vi "robot - Tangent Points.vi"(9 "Diameter":dbl, 10 "Rotation":dbl, 11 "Center Point":cluster{"X":dbl, "Y":dbl}) -> (2 "Second Point":cluster{"X":dbl, "Y":dbl}, 3 "First Point":cluster{"X":dbl, "Y":dbl})   [LabVIEW 2016]
doc: "This VI returns the two points at which a diameter perpendicular to the radius at the given angle (in radians) meet the circle defined by center and diameter."
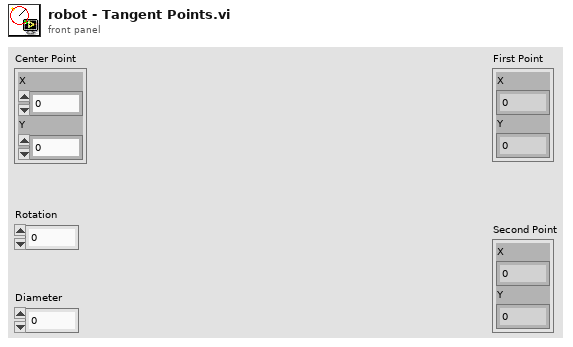
[diagram p1: front panel]
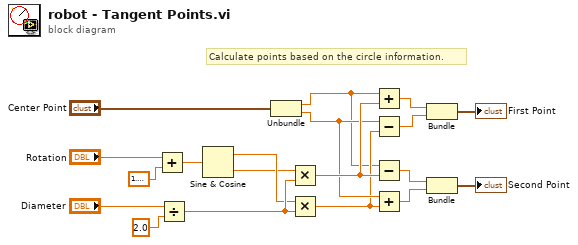
[diagram p0: block diagram]
diagram:
  # "Calculate points based on the circle information."
  n1 = Add(x="Rotation", y=1.5707963267948966) -> (x+y=w16:dbl)
  n2 = Divide(x="Diameter", y=2.0) -> (x/y=w14:dbl)
  n3 = Sine & Cosine(0:w16) -> (1:w13:dbl, 2:w12:dbl)
  n4 = Unbundle("Center Point") -> ("X"=w1:dbl, "Y"=w4:dbl)
  n5 = Multiply(x=w12, y=w14) -> (x*y=w11:dbl)
  n6 = Multiply(x=w13, y=w14) -> (x*y=w3:dbl)
  n7 = Add(x=w1, y=w11) -> (x+y=w10:dbl)
  n8 = Subtract(x=w4, y=w3) -> (x-y=w9:dbl)
  n9 = Subtract(x=w1, y=w11) -> (x-y=w8:dbl)
  n10 = Add(x=w4, y=w3) -> (x+y=w7:dbl)
  n11 = Bundle(w10, w9) -> (→"First Point":cluster{dbl, dbl})  [unwired: 1 in]
  n12 = Bundle(w8, w7) -> (→"Second Point":cluster{dbl, dbl})  [unwired: 1 in]
